vi "main.vi"() -> ()   [LabVIEW 2023]
uses:
  CONTROLS/states.ctl
panel:
  out "Meldung":string
  out "Enum":T1
  in  "stop":bool
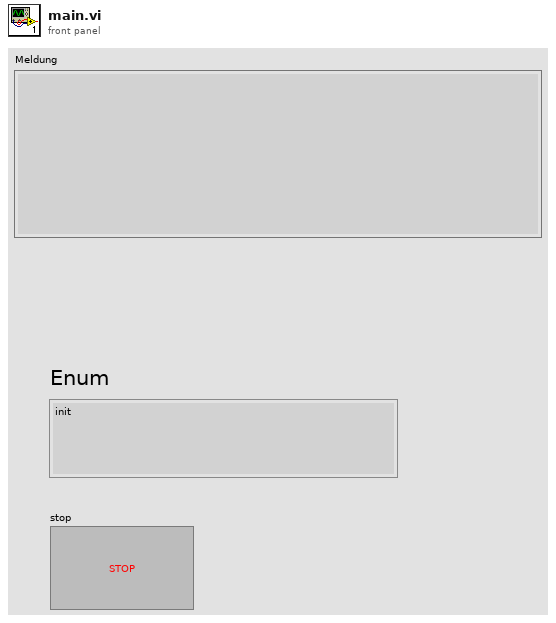
[diagram p1: front panel]
types:
  T1 = typedef "states.ctl" = enum16{"init", "read", "write", "Kundeneingabe", "Betonauswahl", "Bezahlprozeß", "Rechnung", "Zudaten mit Gewichtmessung", "Stop"}
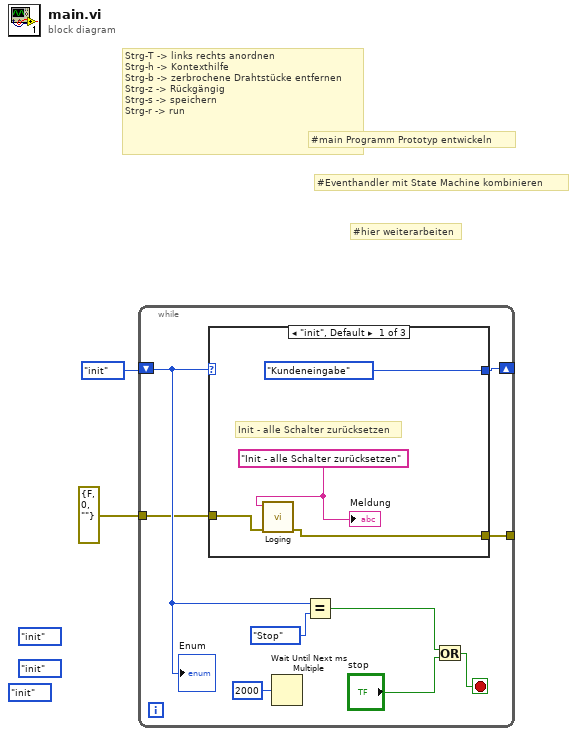
[diagram p0: block diagram]
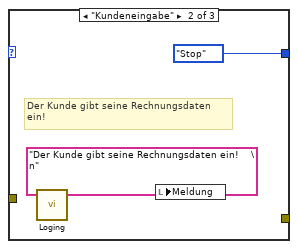
[diagram p2: hidden frame]
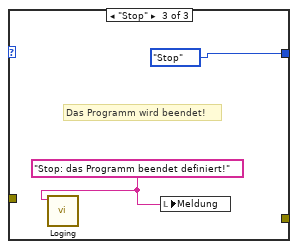
[diagram p3: hidden frame]
diagram:
  (unwired) states."init"
  (unwired) states."init"
  (unwired) states."init"
  # "#hier weiterarbeiten"
  # "#Eventhandler mit State Machine kombinieren"
  # "#main Programm Prototyp entwickeln"
  # "Strg-T -> links rechts anordnen\nStrg-h -> Kontexthilfe\nStrg-b -> zerbrochene Drahtstücke entfernen\nStrg-z -> Rückgängig\nStrg-s -> speichern\nStrg-r -> run"
  n1 = while {
    shift-right: [w11] -> _
    shift-left: states."init" -> [w9]
    tunnel: errorcluster {"status"=FALSE, "code"=0, "source"=""} ("error in") -> [w4]
    tunnel: [w3] -> _
    stop <- w6 stop-if-true
    n2 = case shown="\"init\", Default" w9 {
      tunnel: [states."Kundeneingabe" states."Stop" states."Stop"] -> w11
      tunnel: w4 -> [w13 _ _]
      tunnel: [w12 _ _] -> w3
      frame "init", Default {
        w14 = "Init - alle Schalter zurücksetzen" ("Meldung")
        # "Init - alle Schalter zurücksetzen"
        n3 = call "Loging.vi"("error in"=w13, "log"=w14) -> ("error out"=w12:errorcluster)  [unwired: 9 in]
        "Meldung" <- w14
      }
      frame "Kundeneingabe" {
        w16 = "Der Kunde gibt seine Rechnungsdaten ein!    \n" ("Meldung")
        # "Der Kunde gibt seine Rechnungsdaten \nein!"
        n4 = call "Loging.vi"("log"=w16) -> ()  [unwired: 10 in, 1 out]
        n5 = local write "Meldung"(w16) -> ()
      }
      frame "Stop" {
        w18 = "Stop: das Programm beendet definiert!" ("Meldung")
        # "Das Programm wird beendet!"
        n6 = call "Loging.vi"("log"=w18) -> ()  [unwired: 10 in, 1 out]
        n7 = local write "Meldung"(w18) -> ()
      }
    }
    n8 = Wait Until Next ms Multiple(millisecond multiple=u32 2000) -> ()  [unwired: 1 out]
    n9 = Equal?(x=w9, y=states."Stop") -> (x = y?=w8:bool)
    n10 = Or(x=w8, y="stop") -> (x .or. y?=w6:bool)
    "Enum" <- w9
  }
